vi "Read.ProcessData.vi"(4 "length":i32=-1, 6 "index":i32, 8 "error in (no error)":errorcluster, 10 "timeout ms":i32, 11 "Read in":refnum<class "Read.lvclass">) -> (0 "error out":errorcluster, 1 "Timeout?":bool, 2 "Data":dbl[](array[numeric]), 3 "Read out":refnum<class "Read.lvclass">)   [LabVIEW 2015, in "Data Access Engine.lvlib" / "Read.lvclass"]
uses:
  Read.lvclass
  Read.lvclass/Read.ctl
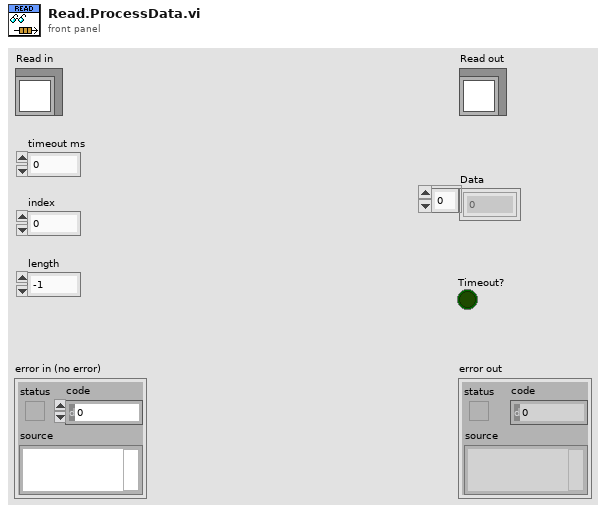
[diagram p1: front panel]
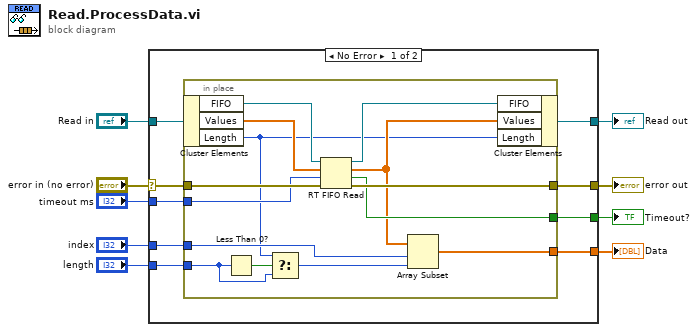
[diagram p0: block diagram]
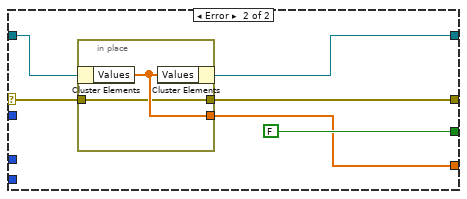
[diagram p2: hidden frame]
diagram:
  n1 = case shown="No Error" "error in (no error)" {
    selector: "error in (no error)" -> [w16 w37]
    tunnel: [w15 w33] -> w8
    tunnel: [w17 w35] -> w6
    tunnel: "Read in" -> [w18 w36]
    tunnel: "timeout ms" -> [w14 _]
    tunnel: [w13 w34] -> w4
    tunnel: [w12 FALSE ("empty?")] -> w3
    tunnel: "length" -> [w11 _]
    tunnel: "index" -> [w10 _]
    frame No Error {
      n2 = in-place {
        in-place-border: w16 -> [w29]
        in-place-border: [w28] -> w15
        in-place-border: w14 -> [w27]
        in-place-border: [w20] -> w13
        in-place-border: [w26] -> w12
        in-place-border: w11 -> [w24]
        in-place-border: w10 -> [w22]
        n3 = in-place-cluster #1(w18) -> ("FIFO"=w32:refnum<k33>, "Values"=w30:dbl[], "Length"=w19:i32)
        n4 = Less Than 0?(x=w24) -> (x < 0?=w25:bool)
        n5 = Select(t=w19, s=w25, f=w24) -> (s? t:f=w23:i32)
        n6 = RT FIFO Read(0:w32, 1:w30, 2:w27, 3:w29) -> (8:w31:refnum<k33>, 9:w21:dbl[], 10:w26:bool, 11:w28:errorcluster)  [unwired: 1 out]
        n7 = Array Subset(array=w21, index=w22, length=w23) -> (w20:dbl[])
        n8 = in-place-cluster #1("FIFO"=w31, "Values"=w21, "Length"=w19) -> (w17:refnum<class "Read.lvclass">)
      }
    }
    frame Error {
      n9 = in-place {
        in-place-border: w37 -> [w39]
        in-place-border: [w39] -> w33
        in-place-border: [w40] -> w34
        n10 = in-place-cluster #2(w36) -> ("Values"=w40:dbl[])
        n11 = in-place-cluster #2("Values"=w40) -> (w35:refnum<class "Read.lvclass">)
      }
    }
  }
  "error out" <- w8
  "Read out" <- w6
  "Data" <- w4
  "Timeout?" <- w3
